vi "MT Demodulate ASK.vi"(0 "input complex waveform":T3={"t0"=0.0, "dt"=1.0, "Y"=[]} {"Y" format="%.3f"; "dt" format="%^.2e"; "t0" format="%.4f"}, 5 "ASK system parameters":T2={"samples per symbol (16)"=16, "symbol map"=[]} {"symbol map" format="%.3f"}, 7 "matched filter coefficients":dbl[](array[numeric]) format="%.2f", 9 "synchronization parameters":T1 {"sync sequence" format="%.2f"}, 11 "error in (no error)":errorcluster, 13 "reset? (T)":bool=TRUE) -> (4 "recovered complex waveform":T3 {"Y" format="%.3f"; "dt" format="%^.2e"; "t0" format="%.4f"}, 6 "output bit stream":i8[](array[numeric]), 8 "measurements":T4 {"phase offset (deg)" format="%.2f"; "frequency drift (Hz)" format="%.2f"; "frequency offset (Hz)" format="%.2f"}, 10 "sync found index (symbols)":dbl format="%.4f", 15 "error out":errorcluster)   [LabVIEW 2020, in "niDMT.lvlib"]
doc: "Demodulates an amplitude shift-keying (ASK)-modulated complex baseband waveform and returns the time-aligned oversampled complex waveform, demodulated bit stream, and results of offset and drift measurements. This VI attempts to remove carrier and phase offset by locking to the carrier signal."
uses:
  <vilib>/addons/Modulation/niDMT.lvlib
  <vilib>/addons/Modulation/Analog/controls/Complex Data Waveform.ctl
  <vilib>/addons/Modulation/Digital/Support/Common/mod_Apply Frequency Offset (Internal).vi
  <vilib>/addons/Modulation/Analog/MT Resample (Complex Cluster).vi
  <vilib>/addons/Modulation/Analog/support/Validators/mod_Fractional Resample Validate.vi
  <vilib>/addons/Modulation/Analog/support/Validators/mod_Check Flush State.vi
  <vilib>/addons/Modulation/Analog/support/mod_FractionalResampler.vi
  <vilib>/addons/Modulation/Analog/support/mod_Integer Rate Interpolation.vi
  <vilib>/addons/Modulation/Analog/support/Validators/mod_Validate Complex Waveform.vi
  <vilib>/addons/Modulation/Analog/support/mod_PerformResampling.vi
  <vilib>/addons/Modulation/Analog/support/Validators/mod_WFErrorHandler.vi
  <vilib>/addons/Modulation/Digital/Support/Common/mod_Truncate FIR Filter (complex).vi
  <vilib>/Utility/error.llb/Error Cluster From Error Code.vi
  <vilib>/addons/Modulation/Analog/support/mod_Resampling Factors.vi
  <vilib>/addons/Modulation/Analog/support/mod_ResamplingFilter.vi
  <vilib>/addons/Modulation/Analog/support/mod_Generate Integer Interpolation Filter.vi
  <vilib>/addons/Modulation/niAMT.lvlib
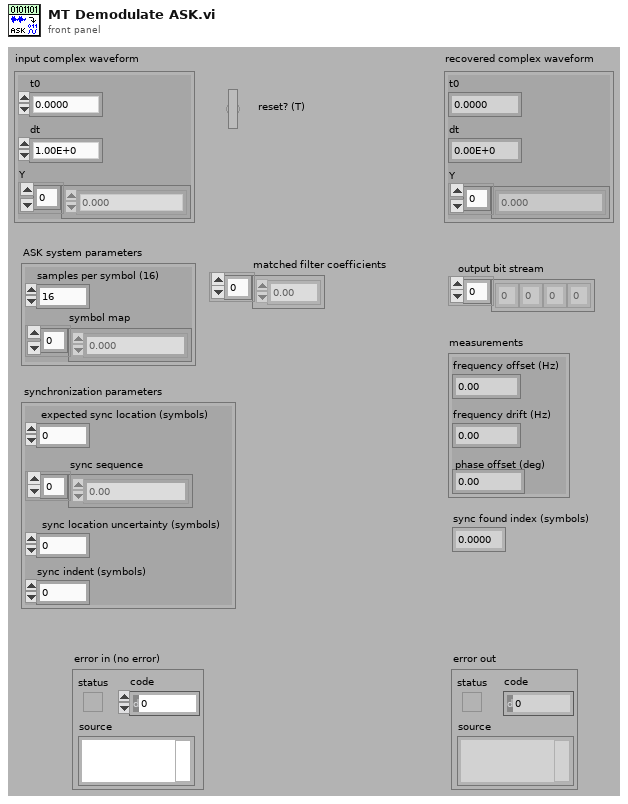
[diagram p1: front panel]
types:
  T1 = cluster{"expected sync location (symbols)":i32, "sync sequence":cdb[], "sync location uncertainty (symbols)":i32, "sync indent (symbols)":i32}
  T2 = cluster{"samples per symbol (16)":i32, "symbol map":cdb[]}
  T3 = typedef "niAMT.lvlib/Complex Data Waveform.ctl" = cluster{"t0":dbl, "dt":dbl, "Y":cdb[]}
  T4 = cluster{"frequency offset (Hz)":dbl, "frequency drift (Hz)":dbl, "phase offset (deg)":dbl}
  T5 = enum16{"FSK", "PSK", "QAM", "MSK", "PAM", "ASK", "CPM"}
  T6 = cluster{dbl, "Frequency Drift, Hz":dbl, "Phase Error Estimate, rads":dbl}
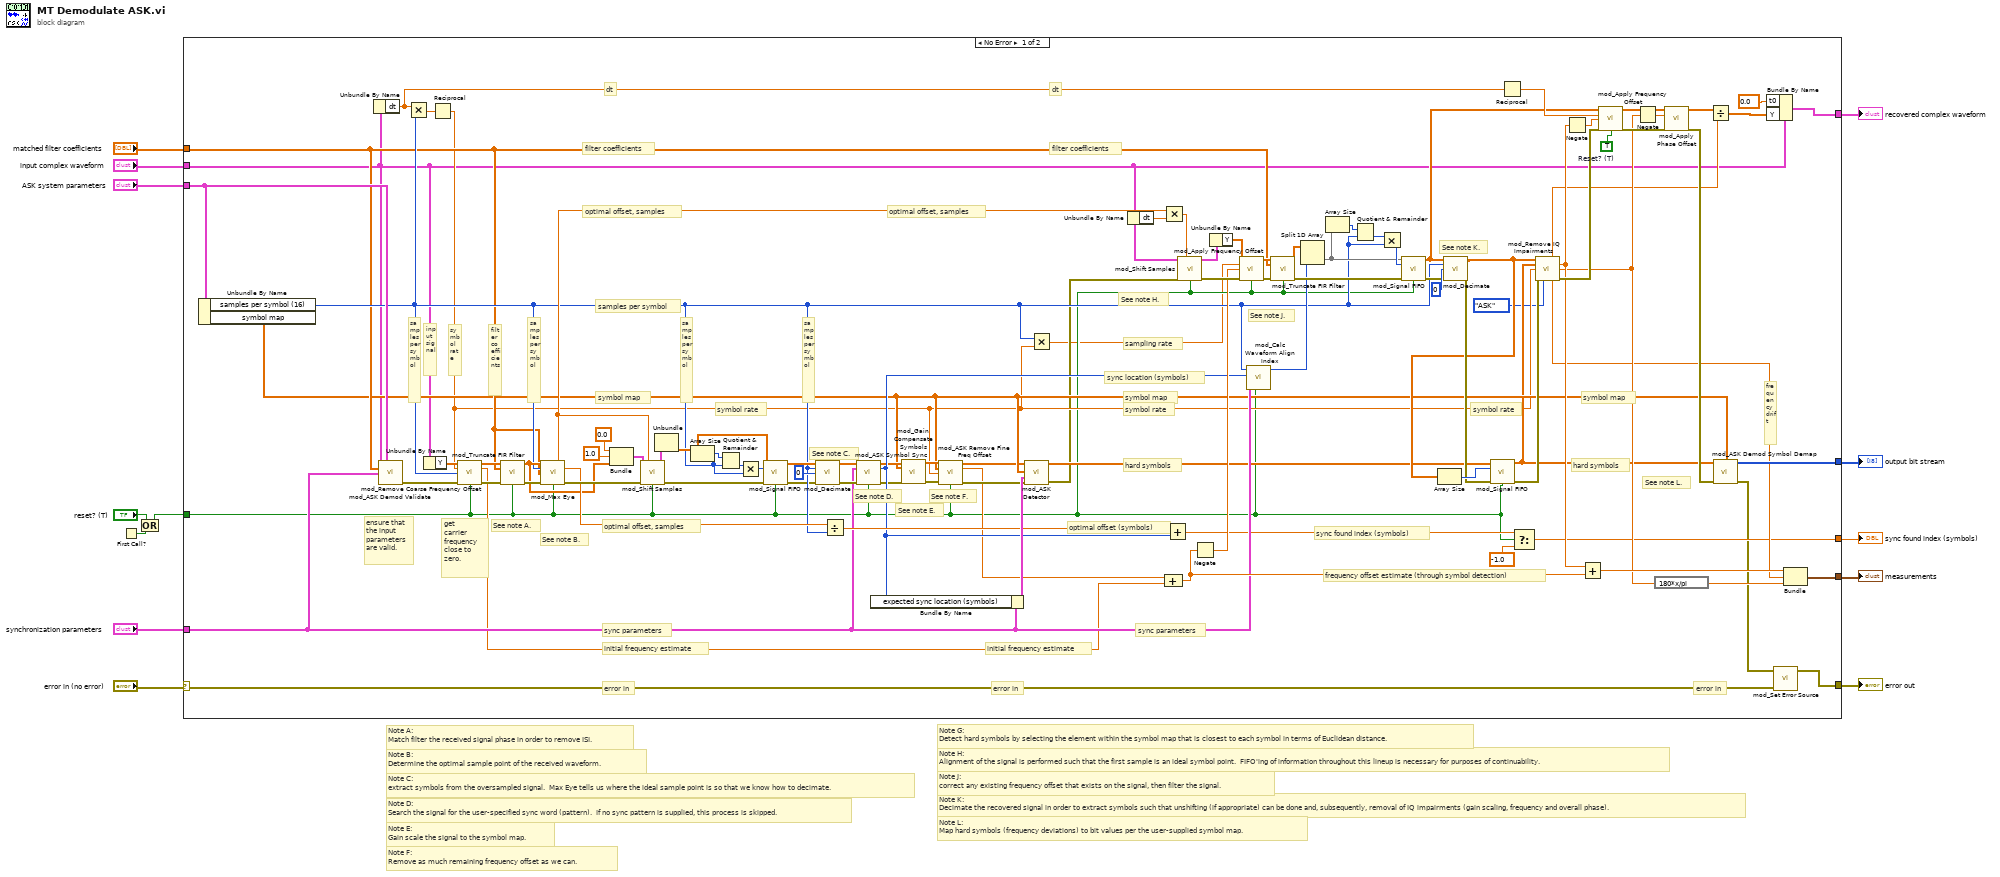
[diagram p0: block diagram]
diagram:
  # "Note E:\nGain scale the signal to the symbol map."
  # "Note L:\nMap hard symbols (frequency deviations) to bit values per the user-supplied symbol map."
  # "Note H:\nAlignment of the signal is performed such that the first sample is an ideal symbol point.  FIFO'ing of information throughout this lineup is necessary for purposes of continuability."
  # "Note D:\nSearch the signal for the user-specified sync word (pattern).  If no sync pattern is supplied, this process is skipped."
  # "Note F:\nRemove as much remaining frequency offset as we can."
  # "Note C:\nextract symbols from the oversampled signal.  Max Eye tells us where the ideal sample point is so that we know how to decimate."
  # "Note B:\nDetermine the optimal sample point of the received waveform."
  # "Note A:\nMatch filter the received signal phase in order to remove ISI."
  # "Note G:\nDetect hard symbols by selecting the element within the symbol map that is closest to each symbol in terms of Euclidean distance."
  # "Note J:\ncorrect any existing frequency offset that exists on the signal, then filter the signal."
  # "Note K:\nDecimate the recovered signal in order to extract symbols such that unshifting (if appropriate) can be done and, subsequently, removal of IQ impairments (gain scaling, frequency and overall phase)."
  n1 = First Call?() -> (First Call?: T/F=w3:bool)
  n2 = Or(x="reset? (T)", y=w3) -> (x .or. y?=w2:bool)
  n3 = case shown="No Error" "error in (no error)" {
    selector: "error in (no error)" -> [w33 w112]
    tunnel: w2 -> [w18 _]
    tunnel: "input complex waveform" -> [w15 _]
    tunnel: [w32 w112] -> w4
    tunnel: "matched filter coefficients" -> [w31 _]
    tunnel: [w111 _] -> w7
    tunnel: [w61 _] -> w6
    tunnel: [w100 _] -> w8
    tunnel: "ASK system parameters" -> [w90 _]
    tunnel: "synchronization parameters" -> [w68 _]
    tunnel: [w106 _] -> w5
    frame No Error {
      w60 = TRUE  # Reset? (T)
      # "frequency offset estimate (through symbol detection)"
      # "error in"
      # "frequency drift"
      # "sync found index (symbols)"
      # "hard symbols"
      # "symbol map"
      # "symbol rate"
      # "dt"
      # "dt"
      # "filter coefficients"
      # "filter coefficients"
      # "sampling rate"
      # "sync location (symbols)"
      # "symbol rate"
      # "symbol rate"
      # "hard symbols"
      # "symbol map"
      # "sync parameters"
      # "error in"
      # "initial frequency estimate"
      # "initial frequency estimate"
      # "sync parameters"
      # "error in"
      # "samples per symbol"
      # "samples per symbol"
      # "symbol map"
      # "samples per symbol"
      # "input signal"
      # "optimal offset, samples"
      # "samples per symbol"
      # "filter coefficients"
      # "See note E."
      # "See note L."
      # "See note K."
      # "See note J."
      # "See note H."
      # "See note D."
      # "See note F."
      # "See note C."
      # "get\ncarrier\nfrequency \nclose to\nzero."
      # "ensure that\nthe input\nparameters\nare valid."
      # "See note B."
      # "See note A."
      # "optimal offset (symbols)"
      # "samples per symbol"
      # "optimal offset, samples"
      # "optimal offset, samples"
      # "symbol rate"
      n4 = Unbundle By Name(w90) -> ("samples per symbol (16)"=w38:i32, "symbol map"=w25:cdb[])
      n5 = Unbundle By Name(w15) -> ("dt"=w86:dbl)
      n6 = call <vilib>:"mod_ASK Demod Validate.vi"("Input Complex Waveform"=w15, "PAM System Parameters"=w90, "Matched Filter Coefficients"=w31, "Synchronization Parameters"=w68) -> ("error out"=w78:errorcluster)  [unwired: 11 out]
      n7 = Multiply(x=w86, y=w38) -> (x*y=w87:dbl)
      n8 = Unbundle By Name(w15) -> ("Y"=w30:cdb[])
      n9 = Reciprocal(x=w87) -> (1/x=w19:dbl)
      n10 = call <vilib>:"mod_Remove Coarse Frequency Offset.vi"("Signal In"=w30, "Symbol Rate, Hz"=w19, "Samples Per Symbol (16)"=w38, "error in (no error)"=w78, "Reset? (T)"=w18) -> ("Signal Out"=w49:cdb[], "Freq Est, Hz"=w56:dbl, "error out"=w108:errorcluster)  [unwired: 8 out]
      n11 = call-poly <vilib>:"mod_Truncate FIR Filter.vi"("Signal In"=w49, "Filter Coefficients"=w31, "error in (no error)"=w108, "Reset? (T)"=w18) -> ("Signal Out"=w47:cdb[], "error out"=w79:errorcluster)  [unwired: 8 in, 2 out]
      n12 = call <vilib>:"mod_Max Eye.vi"("Signal In"=w47, "Samples Per Symbol (16)"=w38, "Filter Coefficients"=w31, "error in (no error)"=w79, "Reset? (T)"=w18) -> ("Waveform Alignment Offset"=w50:dbl, "Optimal Offset (samples)"=w51:dbl, "error out"=w55:errorcluster)  [unwired: 8 out]
      n13 = Bundle(0.0, 1.0, "Signal Out"=w47) -> (w53:cluster{dbl, dbl, "Signal Out":cdb[]})  [unwired: 1 out]
      n14 = call <vilib>:"mod_Shift Samples.vi"("Input Complex Waveform"=w53, "Initial Sample Offset, sec"=w50, "error in (no error)"=w55, "Reset? (T)"=w18) -> ("Output Complex Waveform"=w52:T3, "error out"=w37:errorcluster)  [unwired: 10 in]
      n15 = Unbundle(w52) -> ("Y"=w39:cdb[])  [unwired: 2 out]
      n16 = Array Size(array=w39) -> (size(s)=w41:i32)
      n17 = Quotient & Remainder(x=w41, y=w38) -> (floor(x/y)=w40:i32)  [unwired: 1 out]
      n18 = Multiply(x=w40, y=w38) -> (x*y=w35:i32)
      n19 = call <vilib>:"mod_Signal FIFO.vi"("Signal In"=w39, "Output Length"=w35, "error in (no error)"=w37, "Reset? (T)"=w18) -> ("Signal Out"=w42:cdb[], "error out"=w36:errorcluster)  [unwired: 10 out]
      n20 = call <vilib>:"mod_Decimate.vi"("Signal In"=w42, "Samples Per Symbol (16)"=w38, "Offset"=0, "error in (no error)"=w36) -> ("Signal Out"=w43:cdb[], "error out"=w89:errorcluster)  [unwired: 1 in, 9 out]
      n21 = Divide(x=w51, y=w38) -> (x/y=w84:dbl)
      n22 = call <vilib>:"mod_ASK Symbol Sync.vi"("Signal In"=w43, "Synchronization Parameters"=w68, "error in (no error)"=w89, "Reset? (T)"=w18) -> ("Signal Out"=w27:cdb[], "Sync Location (symbols)"=w67:i32, "error out"=w29:errorcluster)  [unwired: 9 out]
      n23 = Bundle By Name(cluster=w68, "expected sync location (symbols)"=w67) -> (w102:T1)
      n24 = call <vilib>:"mod_Gain Compensate Symbols.vi"("Symbols In"=w27, "Symbol Map"=w25, "error in (no error)"=w29) -> ("Symbols Out"=w26:cdb[], "error out"=w28:errorcluster)  [unwired: 11 out]
      n25 = call <vilib>:"mod_ASK Remove Fine Freq Offset.vi"("Symbols"=w26, "Symbol Map"=w25, "Symbol Rate, Hz"=w19, "error in (no error)"=w28, "Reset? (T)"=w18) -> ("Symbols"=w22:cdb[], "Freq Est, Hz"=w57:dbl, "error out"=w64:errorcluster)  [unwired: 8 out]
      n26 = call <vilib>:"mod_ASK Detector.vi"("Signal In"=w22, "Symbol Map"=w25, "Synchronization Parameters"=w102, "error in (no error)"=w64) -> ("Signal Out"=w65:cdb[], "error out"=w16:errorcluster)  [unwired: 10 out]
      n27 = Multiply(x=w38, y=w19) -> (x*y=w14:dbl)
      n28 = Unbundle By Name(w15) -> ("dt"=w59:dbl)
      n29 = Multiply(x=w50, y=w59) -> (x*y=w103:dbl)
      n30 = Compound Arithmetic op=ADD(w57, w56) -> (w110:dbl)
      n31 = Add(x=w84, y=w67) -> (x+y=w62:dbl)
      n32 = call <vilib>:"mod_Shift Samples.vi"("Input Complex Waveform"=w15, "Initial Sample Offset, sec"=w103, "error in (no error)"=w16, "Reset? (T)"=w18) -> ("Output Complex Waveform"=w105:T3, "error out"=w104:errorcluster)  [unwired: 10 in]
      n33 = Negate(x=w110) -> (-x=w99:dbl)
      n34 = Unbundle By Name(w105) -> ("Y"=w45:cdb[])
      n35 = call <vilib>:"mod_Apply Frequency Offset.vi"("Signal In"=w45, "Rate, pts/sec"=w14, "Freq Offset, Hz"=w99, "error in (no error)"=w104, "Reset? (T)"=w18) -> ("Signal Out"=w109:cdb[], "error out"=w107:errorcluster)  [unwired: 9 out]
      n36 = call <vilib>:"mod_Calc Waveform Align Index.vi"("Reset? (T)"=w18, "Synchronization Parameters"=w68, "Sync Location, symbols"=w67, "Samples Per Symbol (16)"=w38) -> ("align index, samples"=w66:i32)  [unwired: 7 out]
      n37 = call-poly <vilib>:"mod_Truncate FIR Filter.vi"("Signal In"=w109, "Filter Coefficients"=w31, "error in (no error)"=w107, "Reset? (T)"=w18) -> ("Signal Out"=w44:cdb[], "error out"=w74:errorcluster)  [unwired: 8 in, 2 out]
      n38 = Split 1D Array(array=w44, index=w66) -> (second subarray=w48:cdb[])  [unwired: 1 out]
      n39 = Array Size(array=w48) -> (size(s)=w77:i32)
      n40 = Quotient & Remainder(x=w77, y=w38) -> (floor(x/y)=w76:i32)  [unwired: 1 out]
      n41 = Multiply(x=w76, y=w38) -> (x*y=w75:i32)
      n42 = call <vilib>:"mod_Signal FIFO.vi"("Signal In"=w48, "Output Length"=w75, "error in (no error)"=w74, "Reset? (T)"=w18) -> ("Signal Out"=w21:cdb[], "error out"=w73:errorcluster)  [unwired: 10 out]
      n43 = call <vilib>:"mod_Decimate.vi"("Signal In"=w21, "Samples Per Symbol (16)"=w38, "Offset"=0, "error in (no error)"=w73) -> ("Signal Out"=w69:cdb[], "error out"=w71:errorcluster)  [unwired: 1 in, 9 out]
      n44 = Array Size(array=w69) -> (size(s)=w72:i32)
      n45 = call <vilib>:"mod_Signal FIFO.vi"("Signal In"=w65, "Output Length"=w72, "error in (no error)"=w71, "Reset? (T)"=w18) -> ("Signal Out"=w23:cdb[], "error out"=w70:errorcluster)  [unwired: 10 out]
      n46 = Reciprocal(x=w86) -> (1/x=w85:dbl)
      n47 = Select(t=w62, s=w18, f=-1.0) -> (s? t:f=w61:dbl)
      n48 = call <vilib>:"mod_Remove IQ Impairments.vi"("Received Signal In"=w69, "Reference Signal"=w23, "Signal Rate, Hz"=w19, "error in (no error)"=w70, "Modulation Type"=T5."ASK") -> ("Gain Error Estimate"=w81:dbl, "Frequency Estimate, Hz"=w93:dbl, "Phase Error Estimate, rads"=w82:dbl, "Frequency Drift, Hz"=w80:dbl, "error out"=w96:errorcluster)  [unwired: 6 out]
      n49 = Negate(x=w93) -> (-x=w92:dbl)
      n50 = Add(x=w93, y=w110) -> (x+y=w101:dbl)
      n51 = call <vilib>:"mod_Apply Frequency Offset.vi"("Signal In"=w21, "Rate, pts/sec"=w85, "Freq Offset, Hz"=w92, "error in (no error)"=w96, "Reset? (T)"=w60) -> ("Signal Out"=w97:cdb[], "error out"=w95:errorcluster)  [unwired: 9 out]
      n52 = Negate(x=w82) -> (-x=w88:dbl)
      n53 = expression code="180*x/pi"(w82) -> (w83:dbl)
      n54 = call <vilib>:"mod_Apply Phase Offset.vi"("Signal In"=w97, "Phase Offset, rad (0 rad)"=w88, "error in (no error)"=w95) -> ("Signal Out"=w91:cdb[], "error out"=w94:errorcluster)  [unwired: 11 out]
      n55 = Divide(x=w91, y=w81) -> (x/y=w20:cdb[])
      n56 = call <vilib>:"mod_ASK Demod Symbol Demap.vi"("Symbols In"=w23, "Symbol Map"=w25, "error in (no error)"=w94) -> ("Bits Out"=w111:i8[], "error out"=w34:errorcluster)  [unwired: 1 in, 10 out]
      n57 = Bundle By Name(cluster=w15, "t0"=0.0, "Y"=w20) -> (w100:T3)
      n58 = call <vilib>:"mod_Set Error Source.vi"("initial error in (no error)"=w33, "final error in (no error)"=w34) -> ("error out"=w32:errorcluster)  [unwired: 3 out]
      n59 = Bundle(w101, "Frequency Drift, Hz"=w80, "Phase Error Estimate, rads"=w83) -> (w106:T6)  [unwired: 1 out]
    }
    frame Error {
    }
  }
  "error out" <- w4
  "measurements" <- w5
  "sync found index (symbols)" <- w6
  "output bit stream" <- w7
  "recovered complex waveform" <- w8
